vi "TCP.IP Server for Ripple Detection - Experiment 4.vi"() -> ()   [LabVIEW 2021]
doc: "Demonstrates how to set up a basic TCP connection, send data to the specified port once a connection has been established, and terminate the connection once the data has been sent. This VI is designed to stop if the TCP connection is terminated. The data sent in this example is an array of random numbers."
panel:
  out "Iteration terminal":i32
  in  "Stop 2":bool
  in  "File Path":path
  in  "Number of row to read \nat a time":i32=10000
  in  "Client Closed":string="The client VI closed the connection."
  in  "Stop":bool
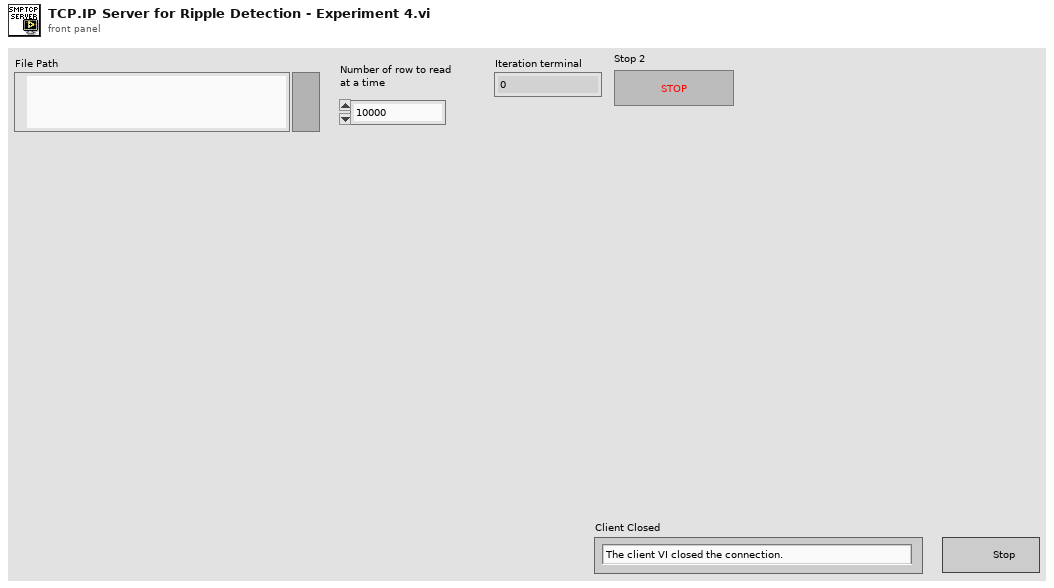
[diagram p1: front panel]
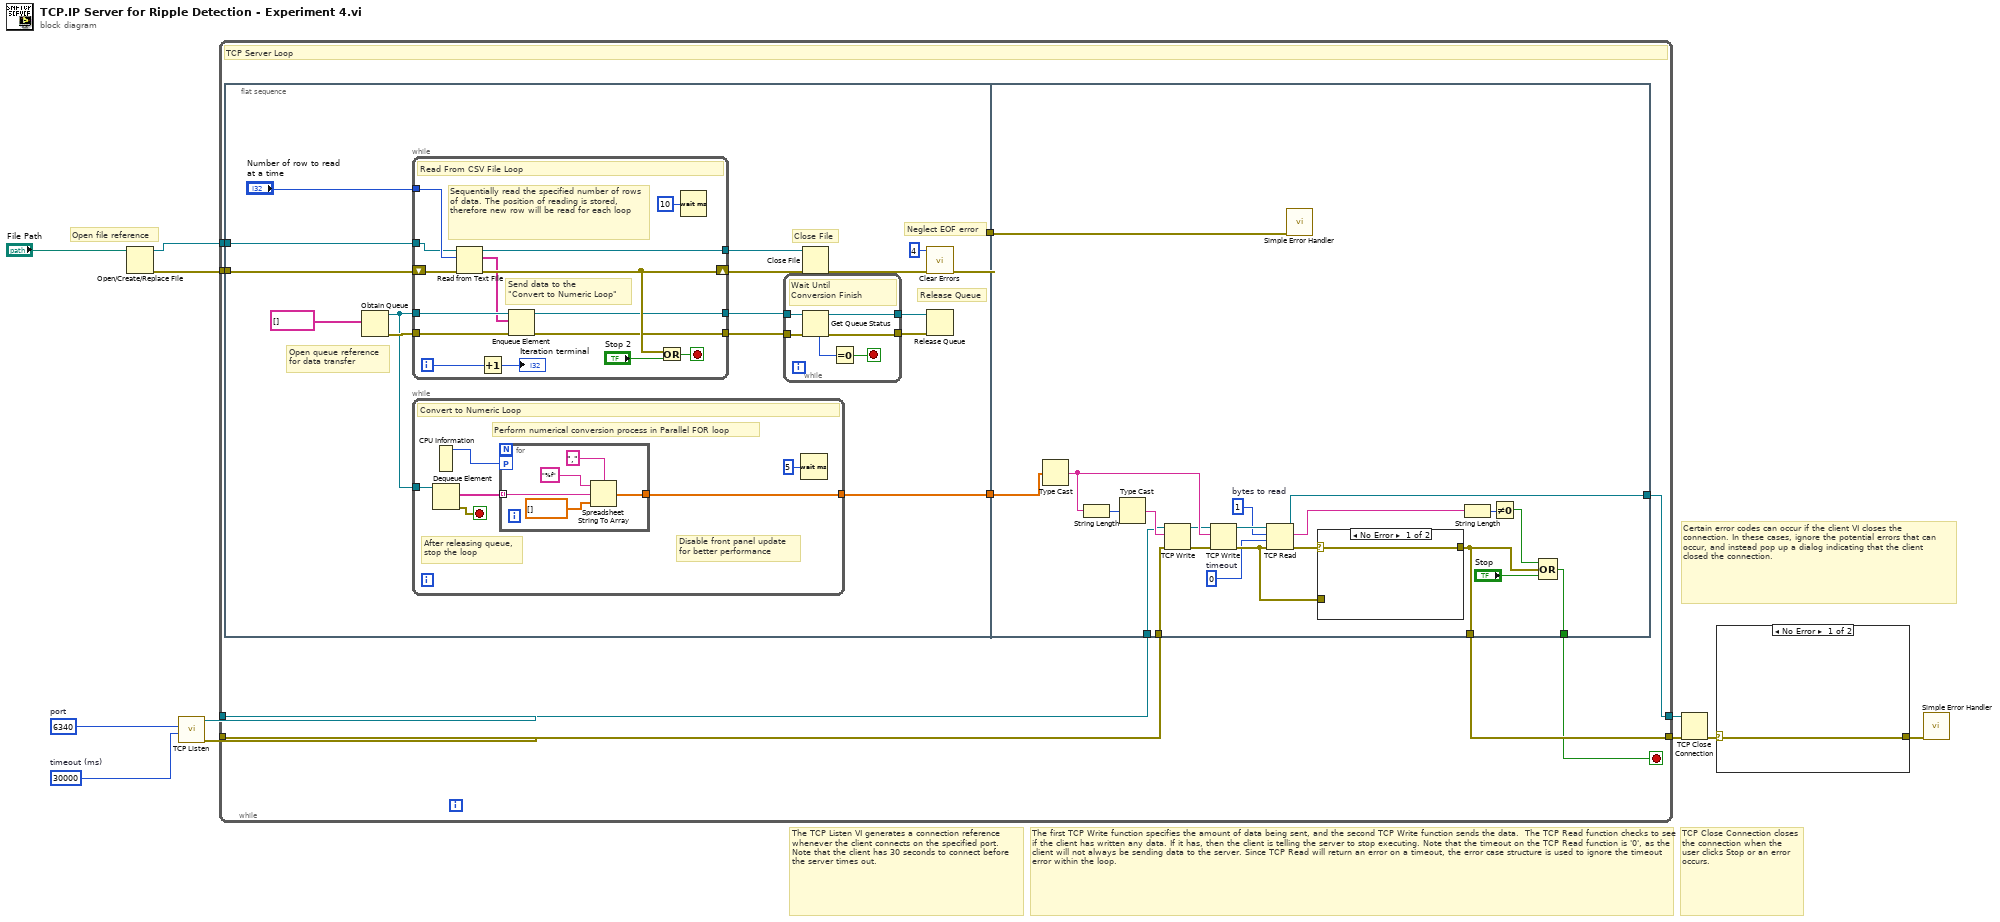
[diagram p0: block diagram]
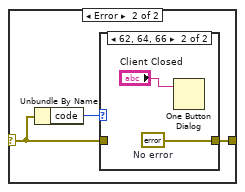
[diagram p2: hidden frame]
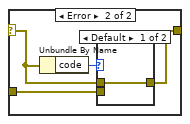
[diagram p4: hidden frame]
diagram:
  w4 = u16 6340  # port
  w5 = 30000  # timeout (ms)
  # "Open file reference"
  # "TCP Close Connection closes the connection when the user clicks Stop or an error occurs."
  # "The TCP Listen VI generates a connection reference whenever the client connects on the specified port. Note that the client has 30 seconds to connect before the server times out."
  # "Certain error codes can occur if the client VI closes the connection. In these cases, ignore the potential errors that can occur, and instead pop up a dialog indicating that the client closed the connection."
  # "The first TCP Write function specifies the amount of data being sent, and the second TCP Write function sends the data.  The TCP Read function checks to see if the client has written any data. If it has, then the client is telling the server to stop executing. Note that the timeout on the TCP Read function is '0', as the client will not always be sending data to the server. Since TCP Read will return an error on a timeout, the error case structure is used to ignore the timeout error within the loop."
  n1 = Open/Create/Replace File(file path (use dialog)="File Path") -> (refnum out=w2:refnum<file>, error out=w1:errorcluster)  [unwired: 5 in, 1 out]
  n2 = call <vilib>:"TCP Listen.vi"("timeout ms (wait forever: -1)"=w5, "port"=w4) -> ("error out"=w6:errorcluster, "connection ID"=w7:refnum<k5>)  [unwired: 5 in, 3 out]
  n3 = while {
    tunnel: [w17] -> w10
    tunnel: [w15] -> w11
    tunnel: w7 -> [w18]
    tunnel: w6 -> [w19]
    tunnel: w2 -> [w13]
    tunnel: w1 -> [w12]
    stop <- w16 stop-if-true
    # "TCP Server Loop"
    n4 = flat-sequence {
      tunnel: [w33] -> w20
      tunnel: [w23] -> w14
      tunnel: w13 -> [w22]
      tunnel: w12 -> [w21]
      tunnel: w20 -> [w89]
      tunnel: w19 -> [w74]
      tunnel: w18 -> [w73]
      tunnel: [w72] -> w17
      tunnel: [w71] -> w16
      tunnel: [w70] -> w15
      tunnel: w14 -> [w69]
      frame #0 {
        # "Neglect EOF error"
        # "Release Queue"
        # "Close File"
        # "Open queue reference\nfor data transfer"
        n5 = Obtain Queue(element data type=string[] [] ("形式文字列")) -> (queue out=w28:refnum<queue>, error out=w29:errorcluster)  [unwired: 4 in, 1 out]
        n6 = while {
          tunnel: [w56] -> w36
          shift-right: [w51] -> w35
          shift-left: w21 -> [w57]
          tunnel: "Number of row to read \nat a time" -> [w52]
          tunnel: w28 -> [w50]
          tunnel: w29 -> [w49]
          tunnel: [w47] -> w27
          tunnel: [w46] -> w26
          tunnel: w22 -> [w43]
          i -> [w54]
          stop <- w55 stop-if-true
          # "Send data to the \n\"Convert to Numeric Loop\""
          # "Sequentially read the specified number of rows of data. The position of reading is stored, therefore new row will be read for each loop"
          # "Read From CSV File Loop"
          n7 = Read from Text File(file (use dialog)=w43, count=w52, error in=w57) -> (refnum out=w56:refnum<file>, text=w48:string[], error out=w51:errorcluster)  [unwired: 1 in, 1 out]
          n8 = Increment(x=w54) -> (x+1=→"Iteration terminal":i32)
          n9 = Enqueue Element(queue=w50, element=w48, error in (no error)=w49) -> (queue out=w47:refnum<queue>, error out=w46:errorcluster)  [unwired: 1 in, 1 out]
          n10 = Or(x=w51, y="Stop 2") -> (x .or. y?=w55:bool)
          n11 = Wait (ms)(milliseconds to wait=u32 10 ("ミリ秒待機時間")) -> ()  [unwired: 1 out]
        }
        n12 = while {
          tunnel: w28 -> [w63]
          tunnel: [w58] -> w23
          stop <- w61 stop-if-true
          # "Disable front panel update \nfor better performance"
          # "After releasing queue,\nstop the loop"
          # "Perform numerical conversion process in Parallel FOR loop"
          # "Convert to Numeric Loop"
          n13 = CPU Information() -> (4:w60:i32)  [unwired: 3 out]
          n14 = Dequeue Element(queue=w63) -> (element=w62:string[], error out=w61:errorcluster)  [unwired: 2 in, 2 out]
          n15 = for "Forループ" {
            tunnel: w62 -> [w65] mode=indexing
            tunnel: [w66] -> w58
            workers-P: w60 -> [_]
            n16 = Spreadsheet String To Array(delimiter (Tab)="," ("デリミタ（タブ）"), format string="%f" ("形式文字列"), spreadsheet string=w65, array type (2D Dbl)=dbl[] []) -> (array=w66:dbl[])
          }
          n17 = Wait (ms)(milliseconds to wait=u32 5 ("ミリ秒待機時間")) -> ()  [unwired: 1 out]
        }
        n18 = while {
          tunnel: w27 -> [w42]
          tunnel: w26 -> [w41]
          tunnel: [w38] -> w24
          tunnel: [w37] -> w25
          stop <- w39 stop-if-true
          # "Wait Until \nConversion Finish"
          n19 = Get Queue Status(queue=w42, error in (no error)=w41) -> (queue out=w38:refnum<queue>, error out=w37:errorcluster, # elements in queue=w40:i32)  [unwired: 1 in, 5 out]
          n20 = Equal To 0?(x=w40) -> (x = 0?=w39:bool)
        }
        n21 = Close File(refnum=w36, error in=w35) -> (error out=w34:errorcluster)  [unwired: 1 out]
        n22 = call <vilib>:"Clear Errors.vi"("error in (no error)"=w34, "specific error code to clear (0: all)"=4) -> ("error out"=w33:errorcluster)  [unwired: 4 in, 1 out]
        n23 = Release Queue(queue=w24, error in (no error)=w25) -> ()  [unwired: 1 in, 3 out]
      }
      frame #1 {
        w76 = 0  # timeout
        w75 = 1  # bytes to read
        n24 = Type Cast(x=w69) -> (*(type *) &x=w81:string)  [unwired: 1 out]
        n25 = String Length(string=w81) -> (length=w79:i32)
        n26 = Type Cast(x=w79) -> (*(type *) &x=w80:string)  [unwired: 1 out]
        n27 = TCP Write(connection ID=w73, data in=w80, error in (no error)=w74) -> (connection ID out=w77:refnum<k5>, error out=w78:errorcluster)  [unwired: 2 out]
        n28 = TCP Write(connection ID=w77, data in=w81, error in (no error)=w78) -> (connection ID out=w83:refnum<k5>, error out=w88:errorcluster)  [unwired: 2 out]
        n29 = TCP Read(connection ID=w83, bytes to read=w75, error in (no error)=w88, 9:w76) -> (connection ID out=w70:refnum<k5>, data out=w85:string, error out=w87:errorcluster)  [unwired: 1 out]
        n30 = call <vilib>:"Simple Error Handler.vi"("error in (no error)"=w89) -> ()  [unwired: 4 in, 5 out]
        n31 = case shown="No Error" w87 {
          selector: w87 -> [w90 w93]
          tunnel: [w90 w91] -> w72
          tunnel: w88 -> [_ w92]
          frame No Error {
          }
          frame Error {
            n32 = Unbundle By Name(w93) -> ("code"=w94:i32)
            n33 = case shown="Default" w94 {
              tunnel: w93 -> [w95 _]
              tunnel: w92 -> [_ w96]
              tunnel: [w95 w96] -> w91
              frame Default {
              }
              frame 56 {
              }
            }
          }
        }
        n34 = String Length(string=w85) -> (length=w84:i32)
        n35 = Not Equal To 0?(x=w84) -> (x != 0?=w86:bool)
        n36 = Compound Arithmetic op=OR(w86, w72, "Stop") -> (w71:bool)
      }
    }
  }
  n37 = TCP Close Connection(connection ID=w11, error in (no error)=w10) -> (error out=w9:errorcluster)  [unwired: 2 out]
  n38 = case shown="No Error" w9 {
    selector: w9 -> [w97 w99]
    tunnel: [w97 w98] -> w8
    frame No Error {
    }
    frame Error {
      n39 = Unbundle By Name(w99) -> ("code"=w100:i32)
      n40 = case shown="62, 64, 66" w100 {
        tunnel: w99 -> [w101 _]
        tunnel: [w101 w103] -> w98
        frame Default {
        }
        frame 62, 64, 66 {
          w103 = errorcluster {"status"=FALSE, "code"=0, "source"=""}  # No error
          n41 = One Button Dialog(message="Client Closed") -> ()  [unwired: 1 in, 1 out]
        }
      }
    }
  }
  n42 = call <vilib>:"Simple Error Handler.vi"("error in (no error)"=w8) -> ()  [unwired: 1 in, 8 out]
